vi "Calculation.vi"(8 "error in":errorcluster, 9 "Zone Selector":bool, 10 "Index in":i32, 11 "Zone Setup Array":cluster{"Zone Selector":string, "Timing":dbl}[](array[cluster])) -> (0 "error out":errorcluster, 1 "Index out":i32, 2 "Index out":i32)   [LabVIEW 2013]
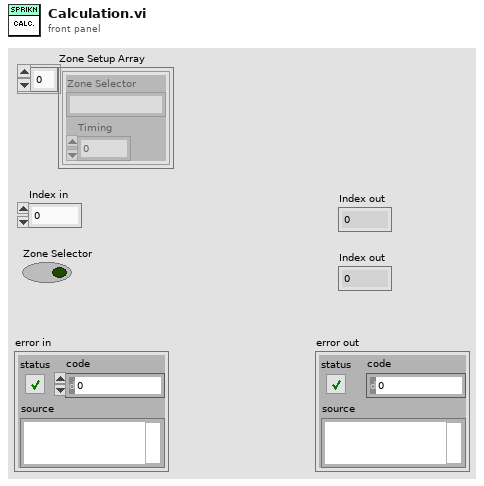
[diagram p1: front panel]
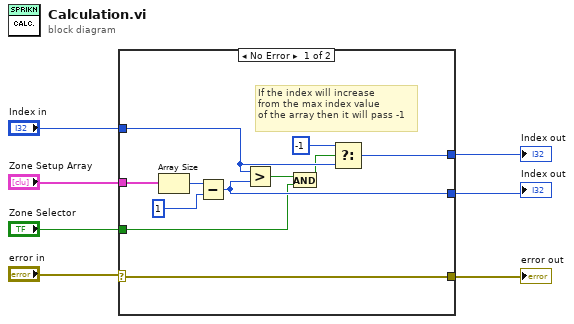
[diagram p0: block diagram]
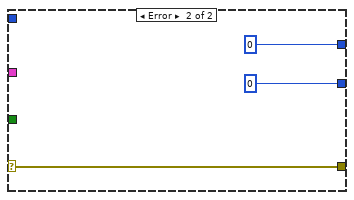
[diagram p2: hidden frame]
diagram:
  n1 = case shown="No Error" "error in" {
    selector: "error in" -> [w8 w21]
    tunnel: [w18 0] -> w7
    tunnel: "Zone Setup Array" -> [w15 _]
    tunnel: "Zone Selector" -> [w14 _]
    tunnel: [w13 0 ("t in")] -> w4
    tunnel: "Index in" -> [w12 _]
    tunnel: [w8 w21] -> w1
    frame No Error {
      # "If the index will increase\nfrom the max index value\nof the array then it will pass -1"
      n2 = Array Size(array=w15) -> (size(s)=w16:i32)
      n3 = Subtract(x=w16, y=1) -> (x-y=w18:i32)
      n4 = Greater?(x=w12, y=w18) -> (0:w9:bool)
      n5 = And(x=w9, y=w14) -> (x .and. y?=w10:bool)
      n6 = Select(t=-1, s=w10, f=w12) -> (s? t:f=w13:i32)
    }
    frame Error {
    }
  }
  "Index out" <- w7
  "Index out" <- w4
  "error out" <- w1
